vi "FTW-ProjectItemManager-CommitChanges.vi"(0 "Project Item Manager":refnum<class "FTW-ProjectItemManager.lvclass">, 11 "error in":errorcluster) -> (4 "Project Item Manager out":refnum<class "FTW-ProjectItemManager.lvclass">, 15 "error out":errorcluster)   [LabVIEW 2012, in "FTW-ProjectItemManager.lvclass"]
doc: "This method takes all properties within the object's Property Bag that are waiting to be written to the Project Item, then writes them as one transaction."
uses:
  FTW-ProjectItemManager.lvclass
panel:
  # "Inputs"
  # "Outputs"
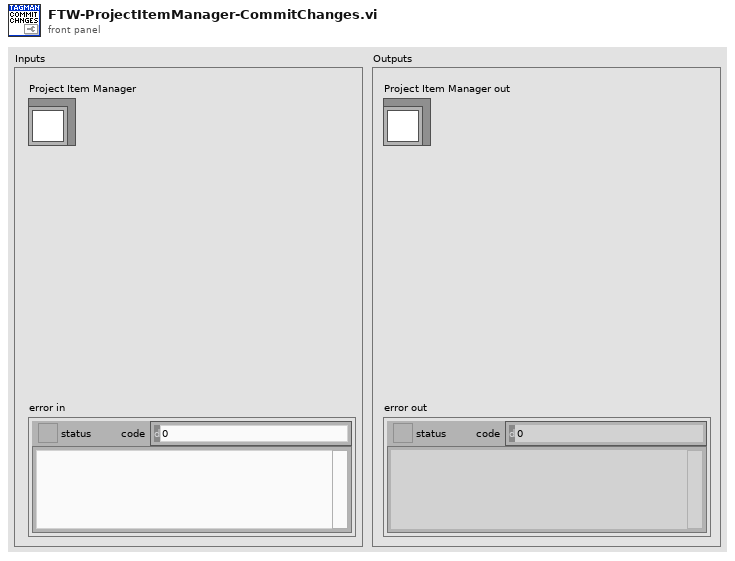
[diagram p1: front panel]
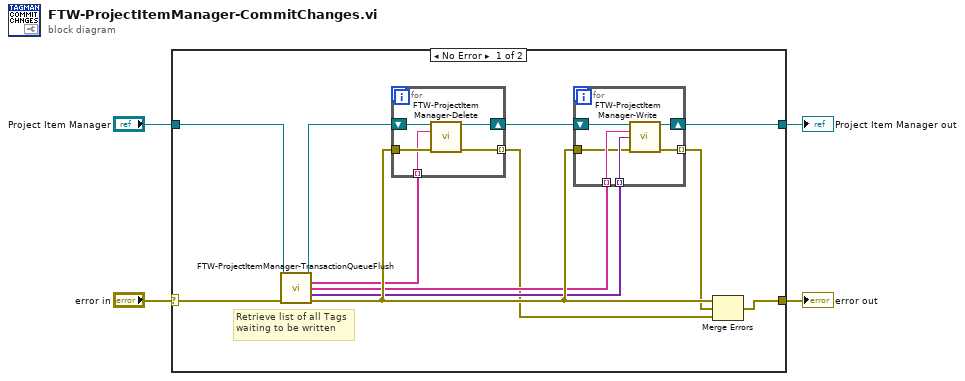
[diagram p0: block diagram]
diagram:
  n1 = case shown="No Error" "error in" {
    selector: "error in" -> [w16 w29]
    tunnel: [w14 w29] -> w4
    tunnel: [w8 w28] -> w2
    tunnel: "Project Item Manager" -> [w15 w28]
    frame No Error {
      # "Retrieve list of all Tags\nwaiting to be written"
      n2 = call "FTW-ProjectItemManager-TransactionQueueFlush.vi"("Project Item Manager"=w15, "error in"=w16) -> ("Project Item Manager out"=w10:refnum<class "FTW-ProjectItemManager.lvclass">, "Remove Transaction Tags Removed"=w5:string[], "Write Transaction Tags Removed"=w12:string[], "Write Transaction Tag Values Removed"=w11:variant[], "error out"=w13:errorcluster)  [unwired: 9 in]
      n3 = for {
        tunnel: [w21] -> w6 mode=indexing
        shift-right: [w19] -> w9
        shift-left: w10 -> [w20]
        tunnel: w13 -> [w18]
        tunnel: w5 -> [w17] mode=indexing
        n4 = call "FTW-ProjectItemManager-Delete.vi"("Project Item Manager"=w20, "Regex Matches to Delete"=w17, "error in"=w18) -> ("Project Item Manager out"=w19:refnum<class "FTW-ProjectItemManager.lvclass">, "error out"=w21:errorcluster)  [unwired: 11 in]
      }
      n5 = for {
        tunnel: [w27] -> w7 mode=indexing
        tunnel: w13 -> [w22]
        tunnel: w12 -> [w26] mode=indexing
        tunnel: w11 -> [w23] mode=indexing
        shift-right: [w24] -> w8
        shift-left: w9 -> [w25]
        n6 = call "FTW-ProjectItemManager-Write.vi"("Project Item Manager"=w25, "Tag"=w26, "Value"=w23, "error in"=w22) -> ("Project Item Manager out"=w24:refnum<class "FTW-ProjectItemManager.lvclass">, "error out"=w27:errorcluster)  [unwired: 10 in]
      }
      n7 = Merge Errors(w13, w7, w6) -> (w14:errorcluster)
    }
    frame Error {
    }
  }
  "error out" <- w4
  "Project Item Manager out" <- w2
